vi "Periodic Tasks.vi"(8 "error for dependency":errorcluster) -> ()   [LabVIEW 2011]
doc: "This VI runs in parallel to other tasks. It can contain as many user-defined periodic loops as you need. These can carry out PID or other sorts of timed response."
uses:
  StateMachineType.ctl
  <vilib>/Rock Robotics/SystemInterfaces/Utilities/FPGA_UtilitiesLED State.ctl
  <vilib>/Rock Robotics/SystemInterfaces/Utilities/FPGA_UtilitiesLED Source.ctl
  Robot Global Data.vi
  <vilib>/addons/control/pid/pid.llb/PID (DBL).vi
  BasketType.ctl
  <vilib>/addons/control/pid/NI_PID_pid.lvlib
panel:
  out "Angle":dbl
  out "Value":i32
  out "Period (sec)":dbl
  in  "Turret Turn output range":cluster{"output high":dbl, "output low":dbl}={"output high"=0.15, "output low"=-0.15} {"output high" min=0.0 max=1.0 step=0.1; "output low" min=-1.0 max=0.0 step=0.1}
  in  "Turret Turn PID gains":T1={"proportional gain (Kc)"=0.4999999999999996, "integral time (Ti, min)"=0.0, "derivative time (Td, min)"=0.0} {"proportional gain (Kc)" step=0.01; "integral time (Ti, min)" step=0.01}
  in  "t":dbl=-0.05
  in  "t 2":dbl=0.05
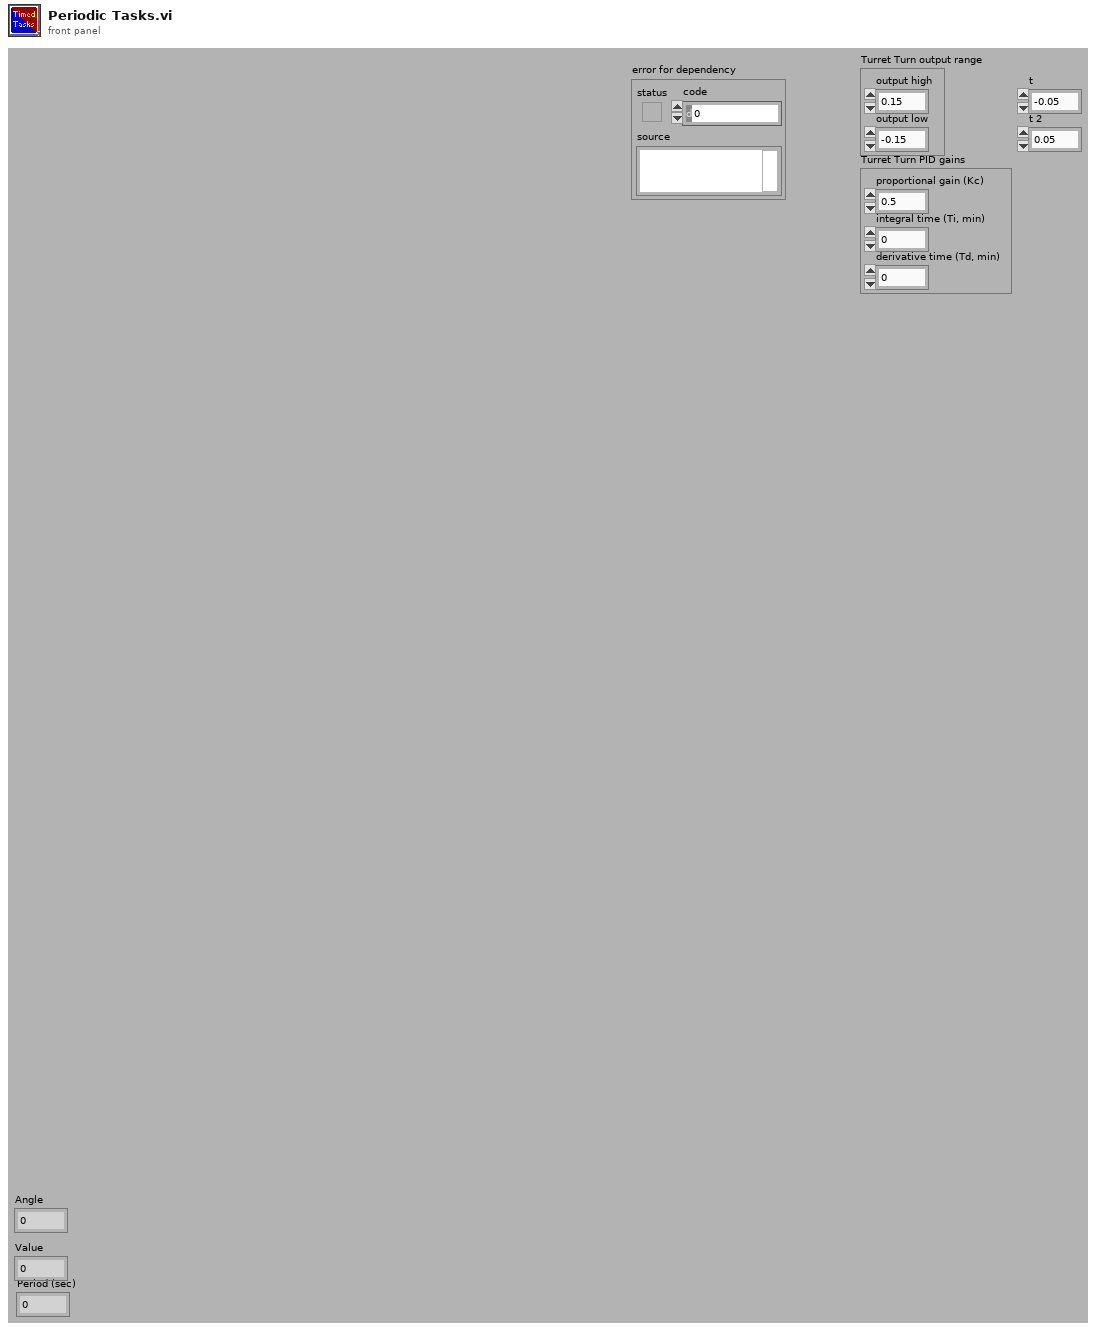
[diagram p1: front panel]
types:
  T1 = cluster{"proportional gain (Kc)":dbl, "integral time (Ti, min)":dbl, "derivative time (Td, min)":dbl}
  T2 = typedef "StateMachineType.ctl" = enum16{"Init", "Idle", "Start", "Do", "Stop"}
  T3 = typedef "WPI_CounterDevRef.ctl" = cluster{"DevStatus":errorcluster, "CntIndex":T4}
  T4 = typedef "FPGA_CounterCtrSystemIndex.ctl" = enum8{"Ctr 0", "Ctr 1", "Ctr 2", "Ctr 3", "Ctr 4", "Ctr 5", "Ctr 6", "Ctr 7", "Invalid"}
  T5 = typedef "WPI_GyroDevRef.ctl" = cluster{"DevStatus":errorcluster, "Analog Module":T6, "Analog Channel":T7, "Offset":dbl, "Gain (VoltsPerDegree/Second)":dbl}
  T6 = typedef "FPGA_TypedefAnalogModule.ctl" = enum16{"Analog Module 1", "Analog Module 2"}
  T7 = typedef "FPGA_AIChannel.ctl" = enum8{"AI 1", "AI 2", "AI 3", "AI 4", "AI 5", "AI 6", "AI 7", "AI 8", "Invalid"}
  T8 = typedef "WPI_EncoderDevRef.ctl" = cluster{"DevStatus":errorcluster, "EncoderIndex":T9, "CounterIndex":T4, "DistancePerCount":dbl, "Decoding Type":T10}
  T9 = typedef "FPGA_EncoderIdx.ctl" = enum8{"Enc 0", "Enc 1", "Enc 2", "Enc 3", "Invalid"}
  T10 = typedef "WPI_EncoderType.ctl" = enum16{"1x", "2x", "4x"}
  T11 = typedef "WPI_MotorControlDeviceRef.ctl" = cluster{"DeviceStatus":errorcluster, "Type":enum16{"PWM", "CAN"}, "PWM":cluster{"Digital Module":T12, "PWM Channel":T13, "DeadBand":T14}, "CAN":cluster{"Device Number":u8, "Control Mode":T15, "Semaphore":T16, "Max Vout":dbl}, "Invert":bool, "TransformRef":T17, "InvTransformRef":T17}
  T12 = typedef "FPGA_TypedefDigitalModule.ctl" = enum16{"Digital Module 1", "Digital Module 2"}
  T13 = typedef "FPGA_DIOPWMChannel.ctl" = enum8{"PWM 1", "PWM 2", "PWM 3", "PWM 4", "PWM 5", "PWM 6", "PWM 7", "PWM 8", "PWM 9", "PWM 10", "Invalid"}
  T14 = typedef "WPI_PWMDeadband.ctl" = cluster{"Name":string, "maxPositivePwm":i32, "minPositivePwm":i32, "centerPwm":i32, "maxNegativePwm":i32, "minNegativePwm":i32, "angularRange":u16}
  T15 = typedef "WPI_CANJaguar_ControlMode.ctl" = enum8{"Percent VBus", "Current", "Speed", "Position", "Voltage"}
  T16 = typedef "Semaphore RefNum" = refnum<k1>
  T17 = typedef "WPI_PWMTransform_ConPane.ctl" = refnum<vi>
  T18 = cluster{"Position":cluster{"X":dbl, "Y":dbl}, "Distance (ft)":dbl}[]
  T19 = cluster{"Position":cluster{"X":dbl, "Y":dbl}, "Distance (ft)":dbl}
  T20 = typedef "FPGA_UtilitiesLED State.ctl" = enum16{"Off", "On", "Toggle"}
  T21 = typedef "FPGA_UtilitiesLED Source.ctl" = enum16{"User LED", "FPGA LED"}
  T22 = typedef "WPI_CompressorDevRef.ctl" = cluster{"DevStatus":errorcluster, "DigitalInputDevRef":T23, "RelayDevRef":T25}
  T23 = typedef "WPI_DigitalInputDevRef.ctl" = cluster{"DevStatus":errorcluster, "DIO Channel":T24, "Digital Module":T12}
  T24 = typedef "FPGA_DIOChannel.ctl" = enum8{"DIO 1", "DIO 2", "DIO 3", "DIO 4", "DIO 5", "DIO 6", "DIO 7", "DIO 8", "DIO 9", "DIO 10", "DIO 11", "DIO 12", "DIO 13", "DIO 14", "Invalid"}
  T25 = typedef "WPI_RelayDevRef.ctl" = cluster{"DevStatus":errorcluster, "Relay Channel":T26, "Digital Module":T12, "Relay Direction":T27}
  T26 = typedef "FPGA_DIORelayChannel.ctl" = enum8{"Relay 1", "Relay 2", "Relay 3", "Relay 4", "Relay 5", "Relay 6", "Relay 7", "Relay 8", "Invalid"}
  T27 = typedef "WPI_RelayDirection.ctl" = enum16{"Both directions", "Forward only", "Reverse only"}
  T28 = typedef "BasketType.ctl" = enum16{"Left", "Bottom", "Right", "Top"}
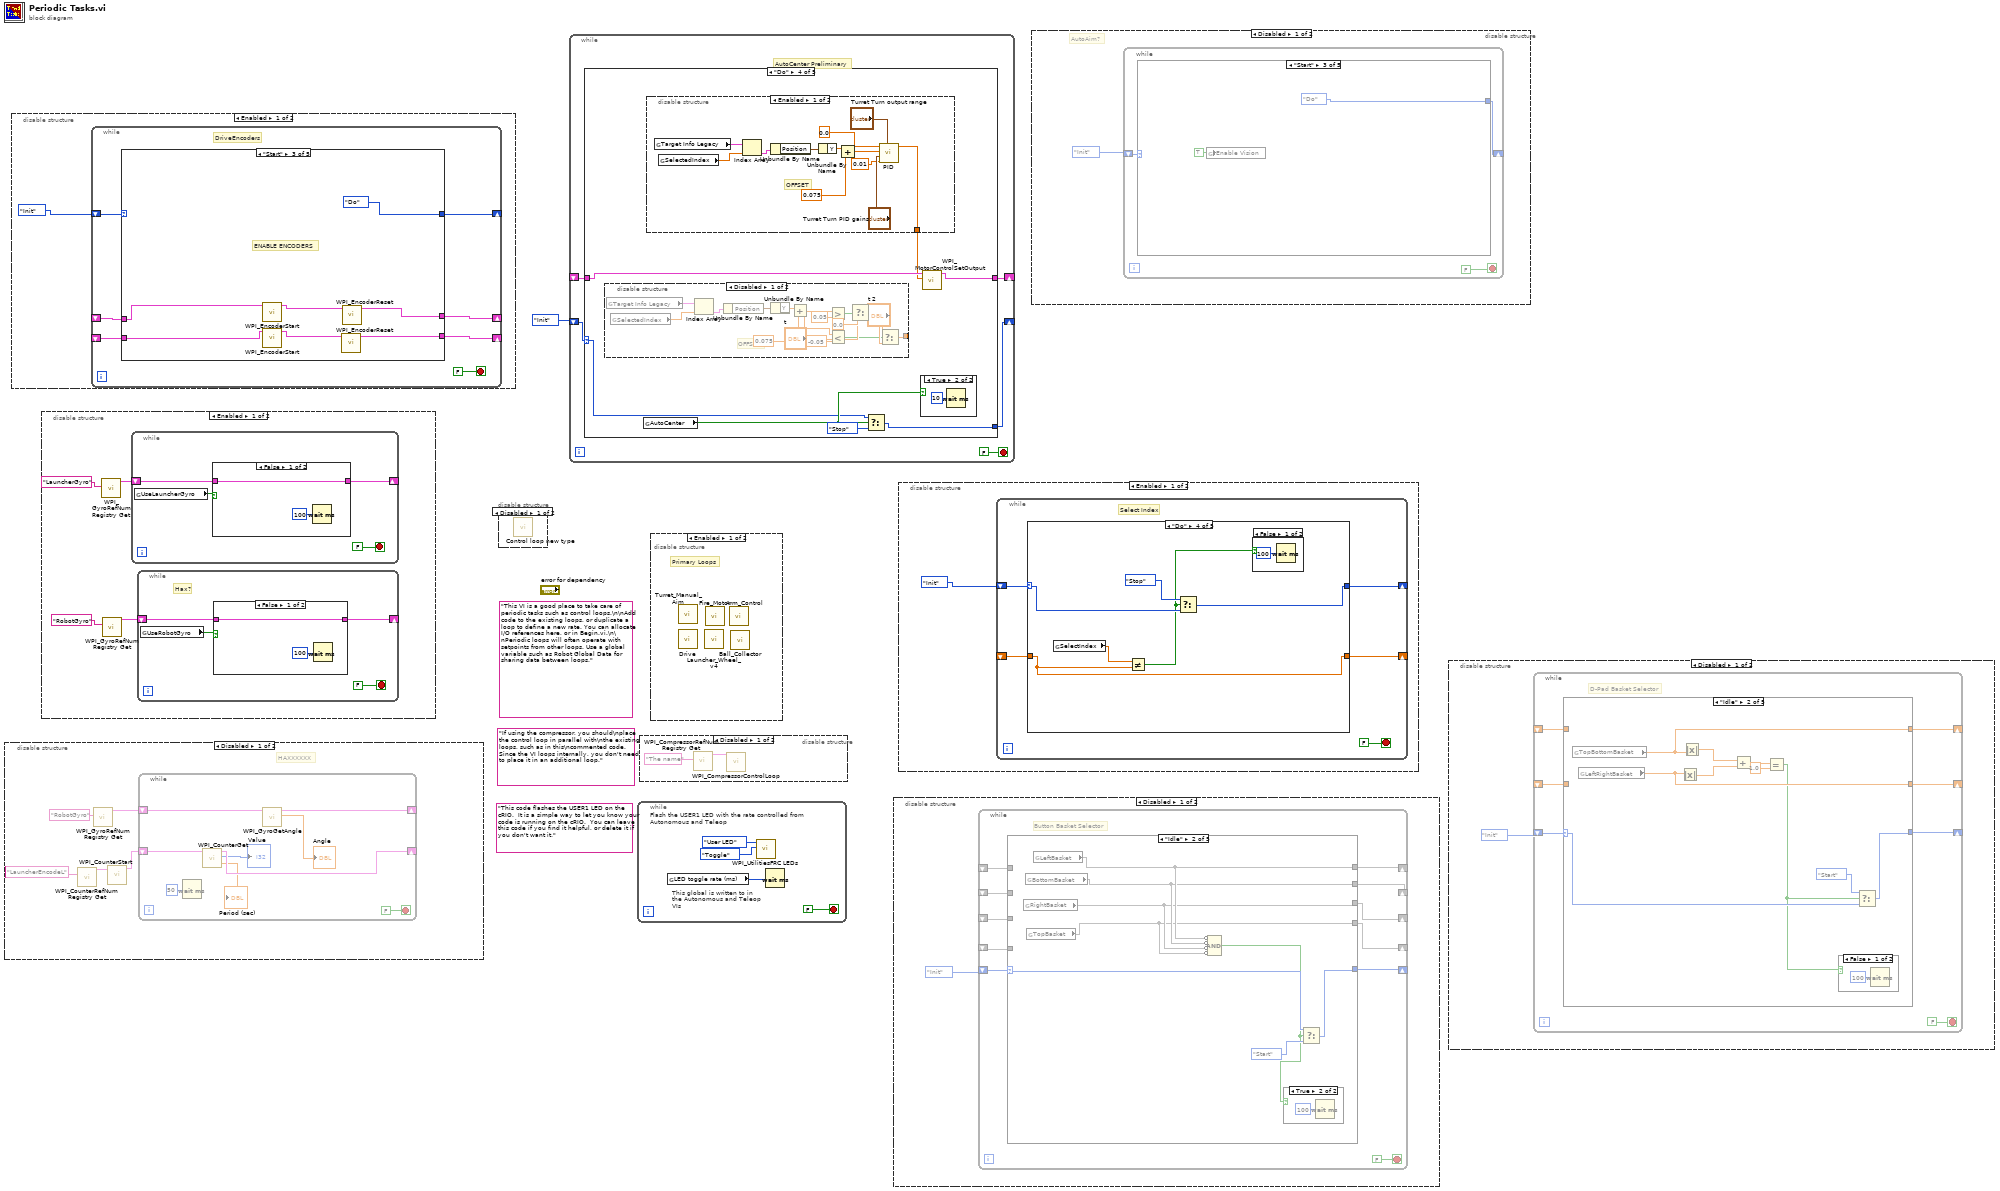
[diagram p0: block diagram]
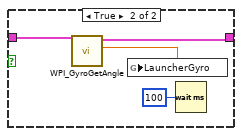
[diagram p3: hidden frame]
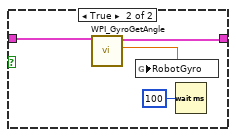
[diagram p4: hidden frame]
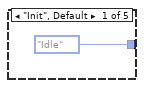
[diagram p6: hidden frame]
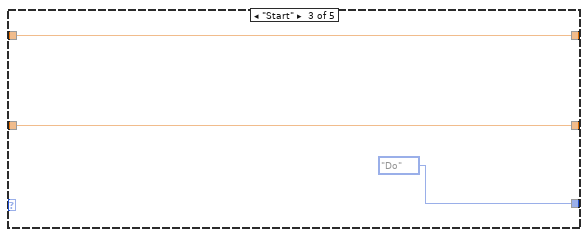
[diagram p8: hidden frame]
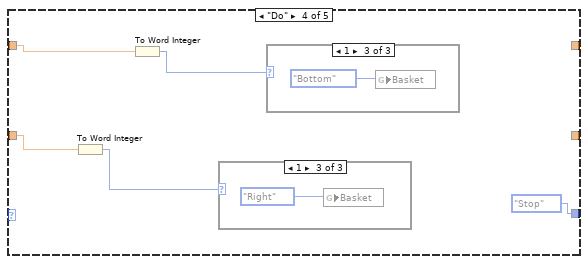
[diagram p9: hidden frame]
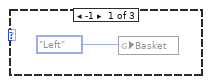
[diagram p10: hidden frame]
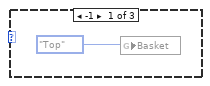
[diagram p12: hidden frame]
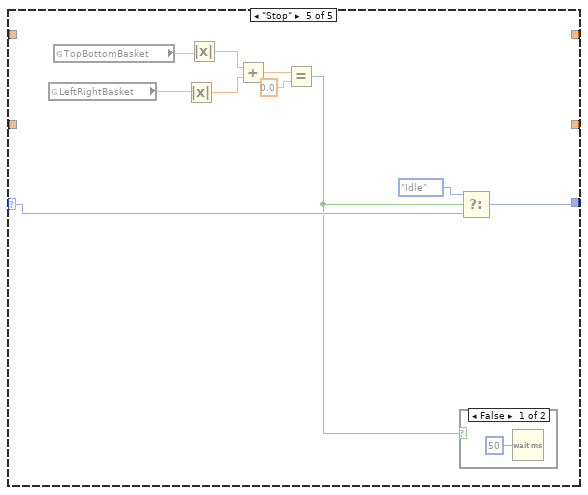
[diagram p14: hidden frame]
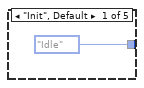
[diagram p17: hidden frame]
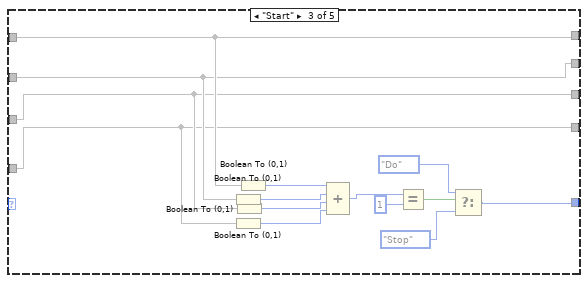
[diagram p19: hidden frame]
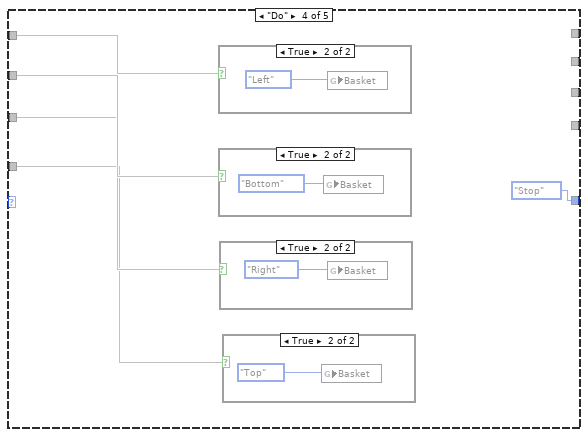
[diagram p20: hidden frame]
diagram:
  (unwired) "This VI is a good place to take care of periodic tasks such as control loops.\n\nAdd code to the existing loops, or duplicate a loop to define a new rate. You can allocate I/O references here, or in Begin.vi.\n\nPeriodic loops will often operate with setpoints from other loops. Use a global variable such as Robot Global Data for sharing data between loops."
  (unwired) "If using the compressor, you should\nplace the control loop in parallel with\nthe existing loops, such as in this\ncommented code. Since the VI loops internally, you don't need to place it in an additional loop."
  (unwired) "This code flashes the USER1 LED on the cRIO.  It is a simple way to let you know your code is running on the cRIO.  You can leave this code if you find it helpful, or delete it if you don't want it."
  n1 = disable-structure shown="Disabled" {
    frame Disabled {
      # "HAXXXXXX"
      n2 = call <vilib>:"WPI_CounterRefNum Registry Get.vi"("refnum name"="LauncherEncodeL") -> ("CounterDevRef"=w3:T3)  [unwired: 9 in, 1 out]
      n3 = call <vilib>:"WPI_GyroRefNum Registry Get.vi"("refnum name"="RobotGyro") -> ("GyroDevRef"=w5:T5)  [unwired: 9 in, 1 out]
      n4 = call <vilib>:"WPI_CounterStart.vi"("CounterDevRef in"=w3) -> ("CounterDevRef out"=w2:T3)  [unwired: 9 in, 1 out]
      n5 = while {
        shift-right: [w14] -> _
        shift-left: w5 -> [w15]
        shift-right: [w9] -> _
        shift-left: w2 -> [w10]
        stop <- FALSE stop-if-true
        n6 = Wait (ms)(milliseconds to wait=u32 50) -> ()  [unwired: 1 out]
        n7 = call <vilib>:"WPI_CounterGet.vi"("CounterDevRef in"=w10) -> ("Value"=→"Value":i32, "CounterDevRef out"=w9:T3, "Period (sec)"=→"Period (sec)":dbl)  [unwired: 5 in, 3 out]
        n8 = call <vilib>:"WPI_GyroGetAngle.vi"("GyroDevRef"=w15) -> ("Angle"=→"Angle":dbl, "GyroDevRef"=w14:T5)  [unwired: 7 in, 2 out]
      }
    }
    frame Enabled {
    }
  }
  n9 = disable-structure shown="Enabled" {
    frame Enabled {
      n10 = while {
        shift-right: [w21] -> _
        shift-left: StateMachineType."Init" -> [w22]
        shift-right: [w20] -> _
        shift-left: _ -> [w17]
        shift-right: [w19] -> _
        shift-left: _ -> [w18]
        stop <- FALSE stop-if-true
        # "DriveEncoders"
        n11 = case shown="\"Start\"" w22 {
          selector: w22 -> [_ w32 _ w63 _]
          tunnel: [StateMachineType."Idle" ("Enum") w31 StateMachineType."Do" ("Enum") w62 StateMachineType."Idle" ("Enum")] -> w21
          tunnel: [w25 w29 w36 w58 w68] -> w20
          tunnel: [w24 w30 w37 w57 w67] -> w19
          tunnel: w18 -> [_ w30 w41 w60 w66]
          tunnel: w17 -> [_ w29 w38 w59 w69]
          frame "Init", Default {
            n12 = call <vilib>:"WPI_EncoderRefNum Registry Get.vi"("refnum name"="DriveEncodeL") -> ("EncoderDevRef"=w24:T8)  [unwired: 9 in, 1 out]
            n13 = call <vilib>:"WPI_EncoderRefNum Registry Get.vi"("refnum name"="DriveEncodeR") -> ("EncoderDevRef"=w25:T8)  [unwired: 9 in, 1 out]
          }
          frame "Idle" {
            n14 = global read "Robot Global Data.vi" "ReadDriveEncoders"() -> (w34:bool)
            n15 = Select(t=StateMachineType."Start" ("Enum"), s=w34, f=w32) -> (s? t:f=w31:T2)
            n16 = case shown="False" w34 {
              frame False {
                n17 = Wait (ms)(milliseconds to wait=u32 100) -> ()  [unwired: 1 out]
              }
              frame True {
              }
            }
          }
          frame "Start" {
            # "ENABLE ENCODERS"
            n18 = call <vilib>:"WPI_EncoderStart.vi"("EncoderDevRef"=w38) -> ("EncoderDevRef"=w39:T8)  [unwired: 9 in, 1 out]
            n19 = call <vilib>:"WPI_EncoderStart.vi"("EncoderDevRef"=w41) -> ("EncoderDevRef"=w40:T8)  [unwired: 9 in, 1 out]
            n20 = call <vilib>:"WPI_EncoderReset.vi"("EncoderDevRef"=w39) -> ("EncoderDevRef"=w36:T8)  [unwired: 9 in, 1 out]
            n21 = call <vilib>:"WPI_EncoderReset.vi"("EncoderDevRef"=w40) -> ("EncoderDevRef"=w37:T8)  [unwired: 9 in, 1 out]
          }
          frame "Do" {
            w48 = -0.5130486441 ("DriveEncoderConstant")
            w51 = 3.141592653589793
            w52 = 180.0 ("y")
            # "CONSTANT: -0.5130486441"
            n22 = global read "Robot Global Data.vi" "ReadDriveEncoders"() -> (w61:bool)
            n23 = call <vilib>:"WPI_EncoderGet.vi"("EncoderDevRef"=w59) -> ("Distance"=w53:dbl, "EncoderDevRef"=w58:T8)  [unwired: 1 in, 8 out]
            n24 = call <vilib>:"WPI_EncoderGet.vi"("EncoderDevRef"=w60) -> ("Distance"=w56:dbl, "EncoderDevRef"=w57:T8)  [unwired: 1 in, 8 out]
            n25 = Divide(x=w56, y=w52) -> (x/y=w55:dbl)
            n26 = Divide(x=w53, y=w52) -> (x/y=w50:dbl)
            n27 = Multiply(x=w50, y=w51) -> (x*y=w49:dbl)
            n28 = Multiply(x=w55, y=w51) -> (x*y=w54:dbl)
            n29 = Multiply(x=w54, y=w48) -> (x*y=w47:dbl)
            n30 = Multiply(x=w49, y=w48) -> (x*y=w46:dbl)
            n31 = Add(x=w47, y=w46) -> (x+y=w45:dbl)
            n32 = Select(t=w63, s=w61, f=StateMachineType."Stop" ("Enum")) -> (s? t:f=w62:T2)
            n33 = case shown="True" w61 {
              frame False {
              }
              frame True {
                n34 = Wait (ms)(milliseconds to wait=u32 50) -> ()  [unwired: 1 out]
              }
            }
            n35 = Divide(x=w45, y=2.0) -> (x/y=w43:dbl)
            n36 = global write "Robot Global Data.vi" "DriveDistance"(w43) -> ()
          }
          frame "Stop" {
            n37 = call <vilib>:"WPI_EncoderStop.vi"("EncoderDevRef"=w66) -> ("EncoderDevRef"=w67:T8)  [unwired: 9 in, 1 out]
            n38 = call <vilib>:"WPI_EncoderStop.vi"("EncoderDevRef"=w69) -> ("EncoderDevRef"=w68:T8)  [unwired: 9 in, 1 out]
          }
        }
      }
    }
    frame Disabled {
    }
  }
  n39 = disable-structure shown="Enabled" {
    frame Enabled {
      n40 = call <vilib>:"WPI_GyroRefNum Registry Get.vi"("refnum name"="LauncherGyro") -> ("GyroDevRef"=w71:T5)  [unwired: 9 in, 1 out]
      n41 = call <vilib>:"WPI_GyroRefNum Registry Get.vi"("refnum name"="RobotGyro") -> ("GyroDevRef"=w73:T5)  [unwired: 9 in, 1 out]
      n42 = while {
        shift-right: [w75] -> _
        shift-left: w71 -> [w76]
        stop <- FALSE stop-if-true
        n43 = global read "Robot Global Data.vi" "UseLauncherGyro"() -> (w77:bool)
        n44 = case shown="False" w77 {
          tunnel: w76 -> [w80 w82]
          tunnel: [w80 w81] -> w75
          frame False {
            n45 = Wait (ms)(milliseconds to wait=u32 100) -> ()  [unwired: 1 out]
          }
          frame True {
            n46 = call <vilib>:"WPI_GyroGetAngle.vi"("GyroDevRef"=w82) -> ("Angle"=w83:dbl, "GyroDevRef"=w81:T5)  [unwired: 7 in, 2 out]
            n47 = global write "Robot Global Data.vi" "LauncherGyro"(w83) -> ()
            n48 = Wait (ms)(milliseconds to wait=u32 100) -> ()  [unwired: 1 out]
          }
        }
      }
      n49 = while {
        shift-right: [w85] -> _
        shift-left: w73 -> [w86]
        stop <- FALSE stop-if-true
        # "Hax?"
        n50 = global read "Robot Global Data.vi" "UseRobotGyro"() -> (w87:bool)
        n51 = case shown="False" w87 {
          tunnel: w86 -> [w90 w92]
          tunnel: [w90 w91] -> w85
          frame False {
            n52 = Wait (ms)(milliseconds to wait=u32 100) -> ()  [unwired: 1 out]
          }
          frame True {
            n53 = call <vilib>:"WPI_GyroGetAngle.vi"("GyroDevRef"=w92) -> ("Angle"=w93:dbl, "GyroDevRef"=w91:T5)  [unwired: 7 in, 2 out]
            n54 = global write "Robot Global Data.vi" "RobotGyro"(w93) -> ()
            n55 = Wait (ms)(milliseconds to wait=u32 100) -> ()  [unwired: 1 out]
          }
        }
      }
    }
    frame Disabled {
    }
  }
  n56 = disable-structure shown="Disabled" {
    frame Disabled {
      n57 = call "Control loop new type.vi"() -> ()  [unwired: 11 in, 1 out]
    }
    frame Enabled {
    }
  }
  n58 = while {
    shift-right: [w98] -> _
    shift-left: StateMachineType."Init" -> [w99]
    shift-right: [w96] -> _
    shift-left: _ -> [w95]
    stop <- FALSE stop-if-true
    # "AutoCenter Preliminary"
    n59 = case shown="\"Do\"" w99 {
      selector: w99 -> [_ w107 w112 w121 _]
      tunnel: [StateMachineType."Idle" w106 w110 w119 StateMachineType."Idle" ("f")] -> w98
      tunnel: [w100 w103 w114 w117 w153] -> w96
      tunnel: w95 -> [_ w103 w114 w118 w154]
      frame "Init", Default {
        n60 = call <vilib>:"WPI_MotorControlRefNum Registry Get.vi"("refnum name"="Turret") -> ("MotorControlDevRef"=w100:T11)  [unwired: 9 in, 1 out]
      }
      frame "Idle" {
        n61 = global read "Robot Global Data.vi" "AutoCenter"() -> (w104:bool)
        n62 = Select(t=StateMachineType."Start", s=w104, f=w107) -> (s? t:f=w106:T2)
        n63 = case shown="False" w104 {
          frame False {
            n64 = Wait (ms)(milliseconds to wait=u32 100) -> ()  [unwired: 1 out]
          }
          frame True {
          }
        }
      }
      frame "Start" {
        n65 = global read "Robot Global Data.vi" "LauncherSteer"() -> (w113:dbl)
        n66 = Equal To 0?(x=w113) -> (x = 0?=w109:bool)
        n67 = case shown="False" w109 {
          frame False {
            n68 = Wait (ms)(milliseconds to wait=u32 10) -> ()  [unwired: 1 out]
          }
          frame True {
          }
        }
        n69 = Select(t=StateMachineType."Do", s=w109, f=w112) -> (s? t:f=w110:T2)
      }
      frame "Do" {
        n70 = disable-structure shown="Disabled" {
          disable-tunnel: [w123 _] -> _
          frame Disabled {
            # "OFFSET"
            n71 = global read "Robot Global Data.vi" "Target Info Legacy"() -> (w138:T18)
            n72 = global read "Robot Global Data.vi" "SelectedIndex"() -> (w137:dbl)
            n73 = Index Array(array=w138, index=w137) -> (element=w136:T19)
            n74 = Unbundle By Name(w136) -> ("Position"=w135:cluster{"X":dbl, "Y":dbl})
            n75 = Unbundle By Name(w135) -> ("Y"=w134:dbl)
            n76 = Add(x=w134, y=0.075) -> (x+y=w124:dbl)
            n77 = Greater?(x=w124, y=0.05) -> (0:w127:bool)
            n78 = Less?(x=w124, y=-0.05) -> (x < y?=w126:bool)
            n79 = Select(t="t", s=w127, f=0.0) -> (s? t:f=w129:dbl)
            n80 = Select(t="t 2", s=w126, f=w129) -> (s? t:f=w123:dbl)
          }
          frame Enabled {
          }
        }
        n81 = global read "Robot Global Data.vi" "AutoCenter"() -> (w122:bool)
        n82 = disable-structure shown="Enabled" {
          disable-tunnel: [w139 _] -> w116
          frame Enabled {
            # "OFFSET"
            n83 = global read "Robot Global Data.vi" "Target Info Legacy"() -> (w150:T18)
            n84 = global read "Robot Global Data.vi" "SelectedIndex"() -> (w149:dbl)
            n85 = Index Array(array=w150, index=w149) -> (element=w148:T19)
            n86 = Unbundle By Name(w148) -> ("Position"=w147:cluster{"X":dbl, "Y":dbl})
            n87 = Unbundle By Name(w147) -> ("Y"=w146:dbl)
            n88 = Add(x=w146, y=0.075 ("Turret Turn offset")) -> (x+y=w143:dbl)
            n89 = call-poly <vilib>:"PID.vi"("output range"="Turret Turn output range", "dt (s)"=0.01, "PID gains"="Turret Turn PID gains", "process variable"=w143, "setpoint"=0.0) -> ("output"=w139:dbl)  [unwired: 5 in, 1 out]
          }
          frame Disabled {
          }
        }
        n90 = Select(t=w121, s=w122, f=StateMachineType."Stop") -> (s? t:f=w119:T2)
        n91 = case shown="True" w122 {
          frame False {
          }
          frame True {
            n92 = Wait (ms)(milliseconds to wait=u32 10) -> ()  [unwired: 1 out]
          }
        }
        n93 = call <vilib>:"WPI_MotorControlSetOutput.vi"("Output"=w116, "MotorControlDevRef"=w118) -> ("MotorControlDevRef"=w117:T11)  [unwired: 8 in, 1 out]
      }
      frame "Stop" {
        n94 = call <vilib>:"WPI_MotorControlSetOutput.vi"("Output"=0.0, "MotorControlDevRef"=w154) -> ("MotorControlDevRef"=w153:T11)  [unwired: 8 in, 1 out]
      }
    }
  }
  n95 = while {
    stop <- FALSE stop-if-true
    # "This global is written to in the Autonomous and Teleop VIs"
    # "Flash the USER1 LED with the rate controlled from Autonomous and Teleop"
    n96 = global read "Robot Global Data.vi" "LED toggle rate (ms)"() -> (w156:u32)
    n97 = call <vilib>:"WPI_UtilitiesFRC LEDs.vi"("State"=FPGA_UtilitiesLED_State."Toggle", "LED Type"=FPGA_UtilitiesLED_Source."User LED") -> ()  [unwired: 1 in, 9 out]
    n98 = Wait (ms)(milliseconds to wait=w156) -> ()  [unwired: 1 out]
  }
  n99 = disable-structure shown="Disabled" {
    frame Disabled {
      n100 = call <vilib>:"WPI_CompressorRefNum Registry Get.vi"("refnum name"="The name") -> ("CompressorDevRef"=w161:T22)  [unwired: 9 in, 1 out]
      n101 = call <vilib>:"WPI_CompressorControlLoop.vi"("CompressorDevRef"=w161) -> ()  [unwired: 11 in]
    }
    frame Enabled {
    }
  }
  n102 = disable-structure shown="Enabled" {
    frame Enabled {
      # "Primary Loops"
      n103 = call "Turret_Manual_Aim.vi"() -> ()  [unwired: 12 in]
      n104 = call "Drive.vi"() -> ()  [unwired: 12 in]
      n105 = call "Launcher_Wheel_v4.vi"() -> ()  [unwired: 12 in]
      n106 = call "Fire_Motor.vi"() -> ()  [unwired: 12 in]
      n107 = call "Arm_Control.vi"() -> ()  [unwired: 12 in]
      n108 = call "Ball_Collector.vi"() -> ()  [unwired: 12 in]
    }
    frame Disabled {
    }
  }
  n109 = disable-structure shown="Disabled" {
    frame Disabled {
      n110 = while {
        shift-right: [w172] -> _
        shift-left: StateMachineType."Init" ("Enum") -> [w173]
        shift-right: [w171] -> _
        shift-left: _ -> [w164]
        shift-right: [w170] -> _
        shift-left: _ -> [w165]
        shift-right: [w169] -> _
        shift-left: _ -> [w166]
        shift-right: [w168] -> _
        shift-left: _ -> [w167]
        stop <- FALSE stop-if-true
        # "Button Basket Selector"
        n111 = case shown="\"Idle\"" w173 {
          selector: w173 -> [_ w176 _ _ w210]
          tunnel: [StateMachineType."Idle" ("Enum") w182 w184 StateMachineType."Stop" ("Enum") w209] -> w172
          tunnel: [_ w178 w194 _ _] -> w171
          tunnel: [_ w179 w195 _ _] -> w170
          tunnel: [_ w180 w196 _ _] -> w169
          tunnel: [_ w181 w197 _ _] -> w168
          tunnel: w167 -> [_ _ w197 w201 _]
          tunnel: w166 -> [_ _ w196 w200 _]
          tunnel: w165 -> [_ _ w195 w199 _]
          tunnel: w164 -> [_ _ w194 w198 _]
          frame "Init", Default {
          }
          frame "Idle" {
            n112 = global read "Robot Global Data.vi" "RightBasket"() -> (w179)
            n113 = global read "Robot Global Data.vi" "BottomBasket"() -> (w180)
            n114 = global read "Robot Global Data.vi" "TopBasket"() -> (w178)
            n115 = global read "Robot Global Data.vi" "LeftBasket"() -> (w181)
            n116 = Compound Arithmetic op=AND(invert w181, invert w180, invert w179, invert w178) -> (w175:bool)
            n117 = case shown="True" w175 {
              frame False {
              }
              frame True {
                n118 = Wait (ms)(milliseconds to wait=u32 100) -> ()  [unwired: 1 out]
              }
            }
            n119 = Select(t=w176, s=w175, f=StateMachineType."Start" ("Enum")) -> (s? t:f=w182:T2)
          }
          frame "Start" {
            n120 = Boolean To (0,1)(Boolean=w196) -> (0, 1=w192:i16)
            n121 = Boolean To (0,1)(Boolean=w194) -> (0, 1=w190:i16)
            n122 = Boolean To (0,1)(Boolean=w195) -> (0, 1=w191:i16)
            n123 = Boolean To (0,1)(Boolean=w197) -> (0, 1=w193:i16)
            n124 = Compound Arithmetic op=ADD(w193, w192, w191, w190) -> (w189:i16)
            n125 = Equal?(x=w189, y=i16 1) -> (x = y?=w187:bool)
            n126 = Select(t=StateMachineType."Do" ("Enum"), s=w187, f=StateMachineType."Stop" ("Enum")) -> (s? t:f=w184:T2)
          }
          frame "Do" {
            n127 = case shown="True" w201 {
              frame False {
              }
              frame True {
                n128 = global write "Robot Global Data.vi" "Basket"(BasketType."Left" ("Basket")) -> ()
              }
            }
            n129 = case shown="True" w200 {
              frame False {
              }
              frame True {
                n130 = global write "Robot Global Data.vi" "Basket"(BasketType."Bottom" ("Basket")) -> ()
              }
            }
            n131 = case shown="True" w199 {
              frame False {
              }
              frame True {
                n132 = global write "Robot Global Data.vi" "Basket"(BasketType."Right" ("Basket")) -> ()
              }
            }
            n133 = case shown="True" w198 {
              frame False {
              }
              frame True {
                n134 = global write "Robot Global Data.vi" "Basket"(BasketType."Top" ("Basket")) -> ()
              }
            }
          }
          frame "Stop" {
            n135 = global read "Robot Global Data.vi" "RightBasket"() -> (w212)
            n136 = global read "Robot Global Data.vi" "BottomBasket"() -> (w213)
            n137 = global read "Robot Global Data.vi" "TopBasket"() -> (w211)
            n138 = global read "Robot Global Data.vi" "LeftBasket"() -> (w214)
            n139 = Compound Arithmetic op=AND(invert w214, invert w213, invert w212, invert w211) -> (w207:bool)
            n140 = case shown="False" w207 {
              frame False {
                n141 = Wait (ms)(milliseconds to wait=u32 100) -> ()  [unwired: 1 out]
              }
              frame True {
              }
            }
            n142 = Select(t=StateMachineType."Idle" ("Enum"), s=w207, f=w210) -> (s? t:f=w209:T2)
          }
        }
      }
    }
    frame Enabled {
    }
  }
  n143 = disable-structure shown="Enabled" {
    frame Enabled {
      n144 = while {
        shift-right: [w219] -> _
        shift-left: StateMachineType."Init" -> [w220]
        shift-right: [w218] -> _
        shift-left: _ -> [w217]
        stop <- FALSE stop-if-true
        # "Select Index"
        n145 = case shown="\"Do\"" w220 {
          selector: w220 -> [_ w229 _ w242 _]
          tunnel: [StateMachineType."Idle" ("Enum") w227 StateMachineType."Do" ("Enum") w244 StateMachineType."Idle" ("Enum")] -> w219
          tunnel: [_ w225 w238 w239 _] -> w218
          tunnel: w217 -> [_ _ w238 w239 _]
          frame "Init", Default {
          }
          frame "Idle" {
            n146 = global read "Robot Global Data.vi" "SelectIndex"() -> (w225:dbl)
            n147 = Absolute Value(x=w225) -> (abs(x)=w226:dbl)
            n148 = Equal?(x=1.0, y=w226) -> (x = y?=w223:bool)
            n149 = Select(t=StateMachineType."Start" ("Enum"), s=w223, f=w229) -> (s? t:f=w227:T2)
            n150 = case shown="False" w223 {
              frame False {
                n151 = Wait (ms)(milliseconds to wait=u32 100) -> ()  [unwired: 1 out]
              }
              frame True {
              }
            }
          }
          frame "Start" {
            n152 = global read "Robot Global Data.vi" "SelectedIndex"() -> (w233:dbl)
            n153 = Negate(x=w238) -> (-x=w234:dbl)
            n154 = Add(x=w233, y=w234) -> (x+y=w232:dbl)
            n155 = Less Than 0?(x=w232) -> (x < 0?=w237:bool)
            n156 = Select(t=0.0, s=w237, f=w232) -> (s? t:f=w235:dbl)
            n157 = global write "Robot Global Data.vi" "SelectedIndex"(w235) -> ()
          }
          frame "Do" {
            n158 = global read "Robot Global Data.vi" "SelectIndex"() -> (w241:dbl)
            n159 = Not Equal?(x=w241, y=w239) -> (x != y?=w240:bool)
            n160 = Select(t=StateMachineType."Stop" ("Enum"), s=w240, f=w242) -> (s? t:f=w244:T2)
            n161 = case shown="False" w240 {
              frame False {
                n162 = Wait (ms)(milliseconds to wait=u32 100) -> ()  [unwired: 1 out]
              }
              frame True {
              }
            }
          }
          frame "Stop" {
          }
        }
      }
    }
    frame Disabled {
    }
  }
  n163 = disable-structure shown="Disabled" {
    frame Disabled {
      # "AutoAim?"
      n164 = while {
        shift-right: [w249] -> _
        shift-left: StateMachineType."Init" ("Enum") -> [w250]
        stop <- FALSE stop-if-true
        n165 = case shown="\"Start\"" w250 {
          selector: w250 -> [_ w253 _ w259 _]
          tunnel: [StateMachineType."Idle" ("Enum") w255 StateMachineType."Do" ("Enum") w262 StateMachineType."Idle" ("Enum")] -> w249
          frame "Init", Default {
          }
          frame "Idle" {
            n166 = global read "Robot Global Data.vi" "EnableAim"() -> (w252:bool)
            n167 = case shown="False" w252 {
              frame False {
                n168 = Wait (ms)(milliseconds to wait=u32 100) -> ()  [unwired: 1 out]
              }
              frame True {
              }
            }
            n169 = Select(t=StateMachineType."Start" ("Enum"), s=w252, f=w253) -> (s? t:f=w255:T2)
          }
          frame "Start" {
            n170 = global write "Robot Global Data.vi" "Enable Vision"(TRUE ("Enable Vision")) -> ()
          }
          frame "Do" {
            n171 = global read "Robot Global Data.vi" "EnableAim"() -> (w260:bool)
            n172 = case shown="True" w260 {
              frame False {
              }
              frame True {
                n173 = Wait (ms)(milliseconds to wait=u32 50) -> ()  [unwired: 1 out]
              }
            }
            n174 = Select(t=w259, s=w260, f=StateMachineType."Stop" ("Enum")) -> (s? t:f=w262:T2)
          }
          frame "Stop" {
            n175 = disable-structure shown="Disabled" {
              frame Disabled {
                n176 = global read "Robot Global Data.vi" "TargetDistance"() -> (w267:dbl)
                n177 = Not A Number/Path/Refnum?(number/path/refnum=w267) -> (NaN/Path/Refnum?=w268:bool)
                n178 = case shown="False" w268 {
                  tunnel: [w272 0.0] -> w266
                  tunnel: w267 -> [w269 _]
                  frame False {
                    n179 = Less Than 0?(x=w269) -> (x < 0?=w271:bool)
                    n180 = Select(t=0.0, s=w271, f=w269) -> (s? t:f=w272:dbl)
                  }
                  frame True {
                  }
                }
                n181 = global write "Robot Global Data.vi" "TargetDistance"(w266) -> ()
              }
              frame Enabled {
              }
            }
            n182 = global write "Robot Global Data.vi" "Enable Vision"(FALSE ("Enable Vision")) -> ()
          }
        }
      }
    }
    frame Enabled {
    }
  }
  n183 = disable-structure shown="Disabled" {
    frame Disabled {
      n184 = while {
        shift-right: [w280] -> _
        shift-left: StateMachineType."Init" ("Enum") -> [w281]
        shift-right: [w278] -> _
        shift-left: _ -> [w276]
        shift-right: [w277] -> _
        shift-left: _ -> [w275]
        stop <- FALSE stop-if-true
        # "D-Pad Basket Selector"
        n185 = case shown="\"Idle\"" w281 {
          selector: w281 -> [_ w286 _ _ w315]
          tunnel: [StateMachineType."Idle" ("Enum") w292 StateMachineType."Do" ("Enum") StateMachineType."Stop" ("Enum") w314] -> w280
          tunnel: [_ w289 w295 _ _] -> w278
          tunnel: [_ w288 w294 _ _] -> w277
          tunnel: w276 -> [_ _ w295 w300 _]
          tunnel: w275 -> [_ _ w294 w298 _]
          frame "Init", Default {
          }
          frame "Idle" {
            n186 = global read "Robot Global Data.vi" "TopBottomBasket"() -> (w289:dbl)
            n187 = global read "Robot Global Data.vi" "LeftRightBasket"() -> (w288:dbl)
            n188 = Absolute Value(x=w288) -> (abs(x)=w290:dbl)
            n189 = Absolute Value(x=w289) -> (abs(x)=w291:dbl)
            n190 = Add(x=w291, y=w290) -> (x+y=w285:dbl)
            n191 = Equal?(x=w285, y=1.0) -> (x = y?=w284:bool)
            n192 = case shown="False" w284 {
              frame False {
                n193 = Wait (ms)(milliseconds to wait=u32 100) -> ()  [unwired: 1 out]
              }
              frame True {
              }
            }
            n194 = Select(t=StateMachineType."Start" ("Enum"), s=w284, f=w286) -> (s? t:f=w292:T2)
          }
          frame "Start" {
          }
          frame "Do" {
            n195 = To Word Integer(number=w298) -> (16bit integer=w297:i16)
            n196 = To Word Integer(number=w300) -> (16bit integer=w299:i16)
            n197 = case shown="1" w297 {
              frame -1 {
                n198 = global write "Robot Global Data.vi" "Basket"(BasketType."Left" ("Basket")) -> ()
              }
              frame 0, Default {
              }
              frame 1 {
                n199 = global write "Robot Global Data.vi" "Basket"(BasketType."Right" ("Basket")) -> ()
              }
            }
            n200 = case shown="1" w299 {
              frame -1 {
                n201 = global write "Robot Global Data.vi" "Basket"(BasketType."Top" ("Basket")) -> ()
              }
              frame 0, Default {
              }
              frame 1 {
                n202 = global write "Robot Global Data.vi" "Basket"(BasketType."Bottom" ("Basket")) -> ()
              }
            }
          }
          frame "Stop" {
            n203 = global read "Robot Global Data.vi" "LeftRightBasket"() -> (w307:dbl)
            n204 = global read "Robot Global Data.vi" "TopBottomBasket"() -> (w308:dbl)
            n205 = Absolute Value(x=w307) -> (abs(x)=w311:dbl)
            n206 = Absolute Value(x=w308) -> (abs(x)=w312:dbl)
            n207 = Add(x=w312, y=w311) -> (x+y=w310:dbl)
            n208 = Equal?(x=w310, y=0.0) -> (x = y?=w306:bool)
            n209 = case shown="False" w306 {
              frame False {
                n210 = Wait (ms)(milliseconds to wait=u32 50) -> ()  [unwired: 1 out]
              }
              frame True {
              }
            }
            n211 = Select(t=StateMachineType."Idle" ("Enum"), s=w306, f=w315) -> (s? t:f=w314:T2)
          }
        }
      }
    }
    frame Enabled {
    }
  }
